vi "Obtain Async ACQ Data Notifier.vi"(8 "error in (no error)":errorcluster) -> (0 "error out":errorcluster, 3 "Async ACQ Notifier out":refnum<notifier>)   [LabVIEW 2014, in "WINFAS 2 Data Queue.lvlib"]
uses:
  WINFAS 2 Data Queue.lvlib
  Async Acquisition Data Cluster.ctl
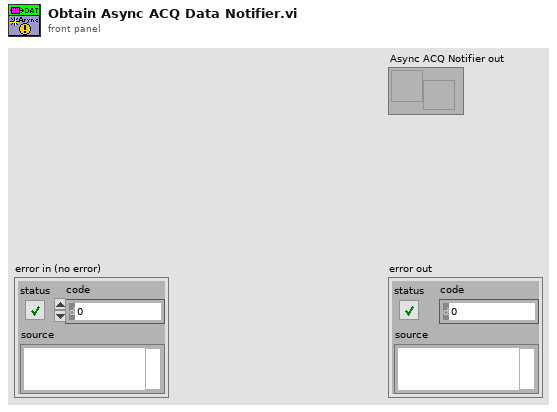
[diagram p1: front panel]
types:
  T1 = typedef "WINFAS 2 Data Queue.lvlib/Async Acquisition Data Cluster.ctl" = cluster{"Data":sgl[]}
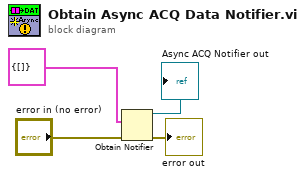
[diagram p0: block diagram]
diagram:
  n1 = Obtain Notifier(notification data type=T1 {"Data"=[]} ("Async ACQ"), error in (no error)="error in (no error)") -> (notifier out=→"Async ACQ Notifier out":refnum<notifier>, error out=→"error out":errorcluster)  [unwired: 2 in, 1 out]
